vi "Clear Trees.vi"(8 "error in (no error)":errorcluster, 11 "SequenceViewPanel in":refnum<class "SequenceViewPanel.lvclass">) -> (0 "error out":errorcluster, 3 "SequenceViewPanel out":refnum<class "SequenceViewPanel.lvclass">)   [LabVIEW 2020, in "TSnax UI.lvlib" / "SequenceViewPanel.lvclass"]
uses:
  SequenceViewPanel.lvclass
  SequenceViewPanel.lvclass/SequenceViewPanel.ctl
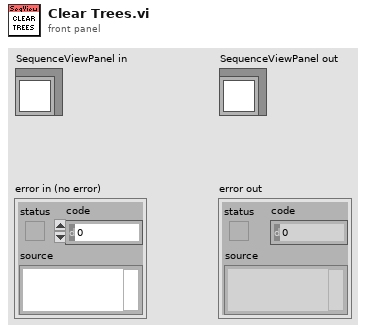
[diagram p1: front panel]
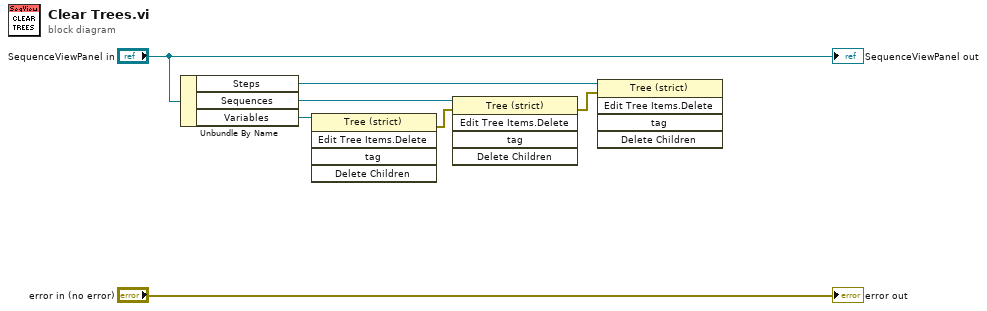
[diagram p0: block diagram]
diagram:
  n1 = Unbundle By Name("SequenceViewPanel in") -> ("Steps"=w2:refnum<vi>, "Sequences"=w4:refnum<vi>, "Variables"=w5:refnum<vi>)
  n2 = invoke class="Tree (strict)" method="Edit Tree Items.Delete"(reference=w5) -> (error out=w3:errorcluster)  [unwired: 4 in, 4 out]
  n3 = invoke class="Tree (strict)" method="Edit Tree Items.Delete"(reference=w4, error in=w3) -> (error out=w1:errorcluster)  [unwired: 3 in, 4 out]
  n4 = invoke class="Tree (strict)" method="Edit Tree Items.Delete"(reference=w2, error in=w1) -> ()  [unwired: 3 in, 5 out]
  "error out" <- "error in (no error)"
  "SequenceViewPanel out" <- "SequenceViewPanel in"
